vi "Obtain.vi"(8 "Error In":errorcluster, 11 "Listener ID":string) -> (0 "Error Out":errorcluster, 3 "Listener":refnum<queue>)   [LabVIEW 2014, in "LV-Logger.lvlib"]
uses:
  LV-Logger.lvlib
  Controls/Message.ctl
  Controls/Level.ctl
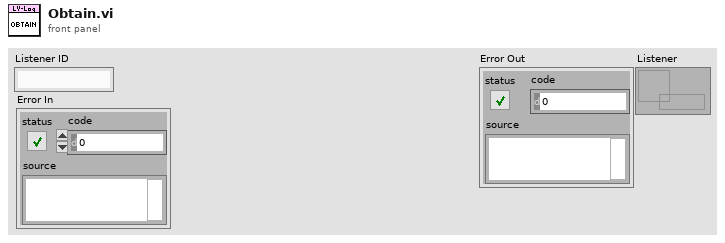
[diagram p1: front panel]
types:
  T1 = typedef "LV-Logger.lvlib/Message.ctl" = cluster{"Time Stamp":timestamp, "Level":T2, "Source":string, "Text":string}
  T2 = typedef "LV-Logger.lvlib/Level.ctl" = enum16{"Fatal", "Error", "Warn", "Info", "Debug", "Trace"}
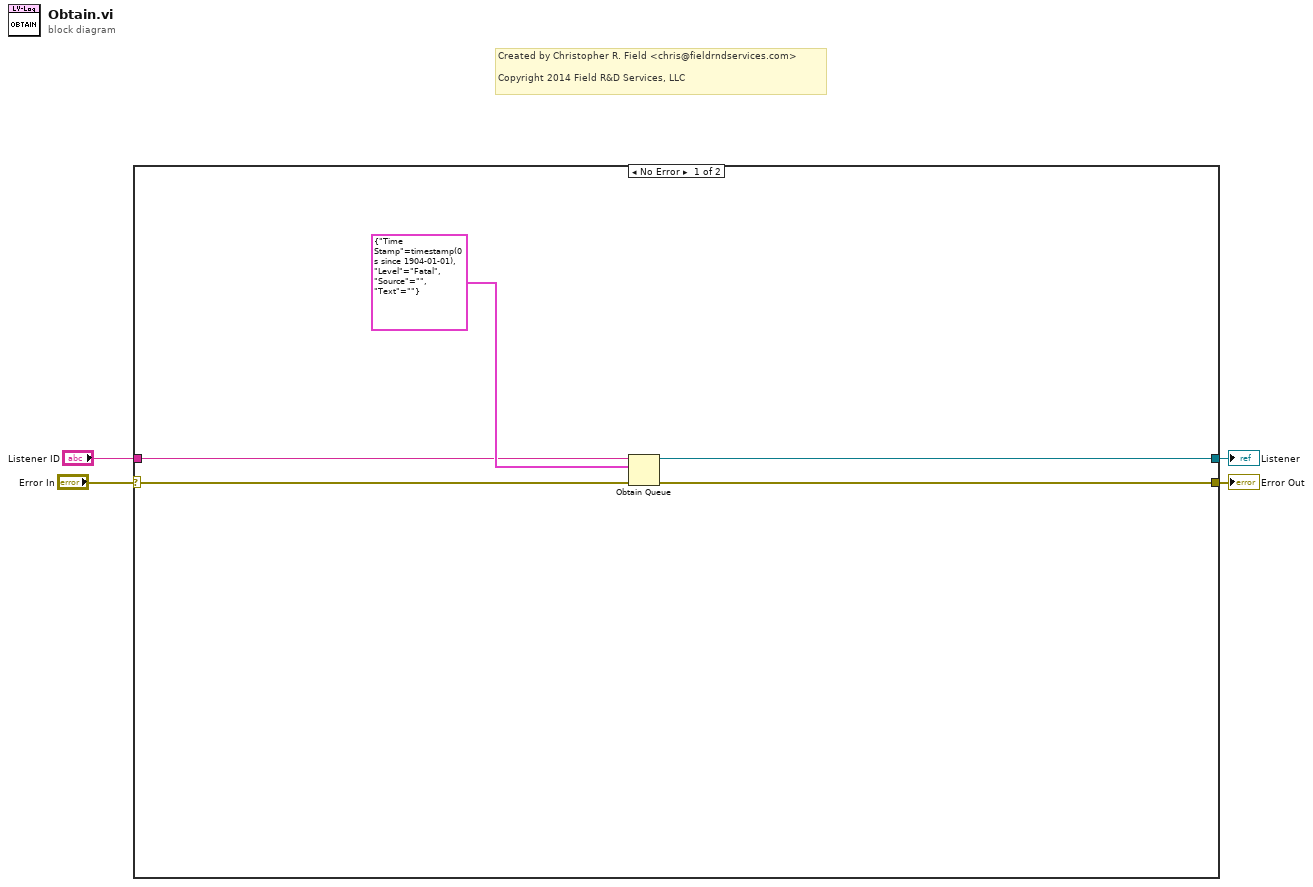
[diagram p0: block diagram]
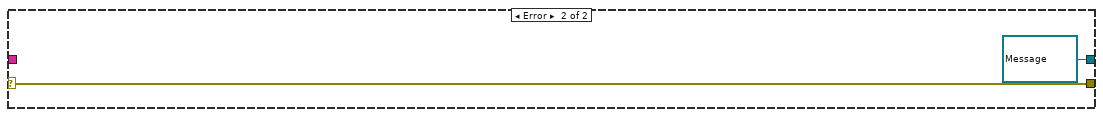
[diagram p2: hidden frame]
diagram:
  # "Created by Christopher R. Field <chris@fieldrndservices.com>\n\nCopyright 2014 Field R&D Services, LLC"
  n1 = case shown="No Error" "Error In" {
    selector: "Error In" -> [w7 w11]
    tunnel: "Listener ID" -> [w8 _]
    tunnel: [w6 w11] -> w2
    tunnel: [w5 refnum<queue> refnum ("queue out")] -> w1
    frame No Error {
      n2 = Obtain Queue(name (unnamed)=w8, element data type=T1 {"Time Stamp"=timestamp(0 s since 1904-01-01), "Level"=enum."Fatal", "Source"="", "Text"=""} ("Message"), error in (no error)=w7) -> (queue out=w5:refnum<queue>, error out=w6:errorcluster)  [unwired: 2 in, 1 out]
    }
    frame Error {
    }
  }
  "Error Out" <- w2
  "Listener" <- w1
